vi "Get Array Size.vi"(8 "error in (no error)":errorcluster, 11 "JSON Value in":refnum<class "JSON Value.lvclass">) -> (0 "error out":errorcluster, 3 "size(s)":i32)   [LabVIEW 2016, in "JSON Value.lvclass"]
doc: "Returns the number of elements in a JSON Array"
uses:
  JSON Value.lvclass
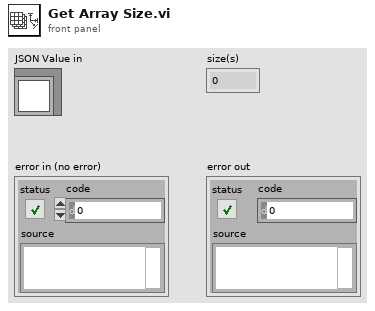
[diagram p1: front panel]
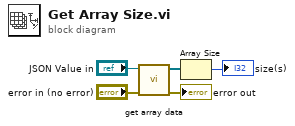
[diagram p0: block diagram]
diagram:
  n1 = call "get array data.vi"("error in (no error)"="error in (no error)", "JSON Value in"="JSON Value in") -> ("error out"=→"error out":errorcluster, "JSON Array out"=w3:refnum<class "JSON Value.lvclass">[])  [unwired: 8 in]
  n2 = Array Size(array=w3) -> (size(s)=→"size(s)":i32)
